vi "DAQ_Readings_from_DVS_plotting_and_saving.vi"() -> ()   [LabVIEW 2013]
uses:
  <vilib>/DAQmx/read.llb/DAQmx Read (Analog DBL 1Chan 1Samp).vi
  <vilib>/Utility/file.llb/Write To Spreadsheet File (string).vi
  <vilib>/DAQmx/miscellaneous.llb/DAQmx Fill In Error Info.vi
panel:
  out "Waveform Chart":cluster{dbl, dbl, dbl, dbl, dbl}(graph)
  in  "stop":bool
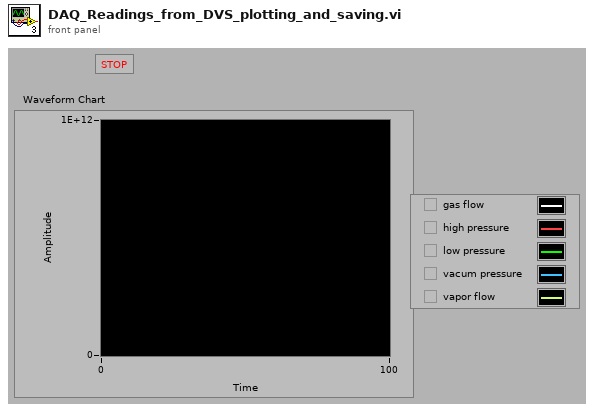
[diagram p1: front panel]
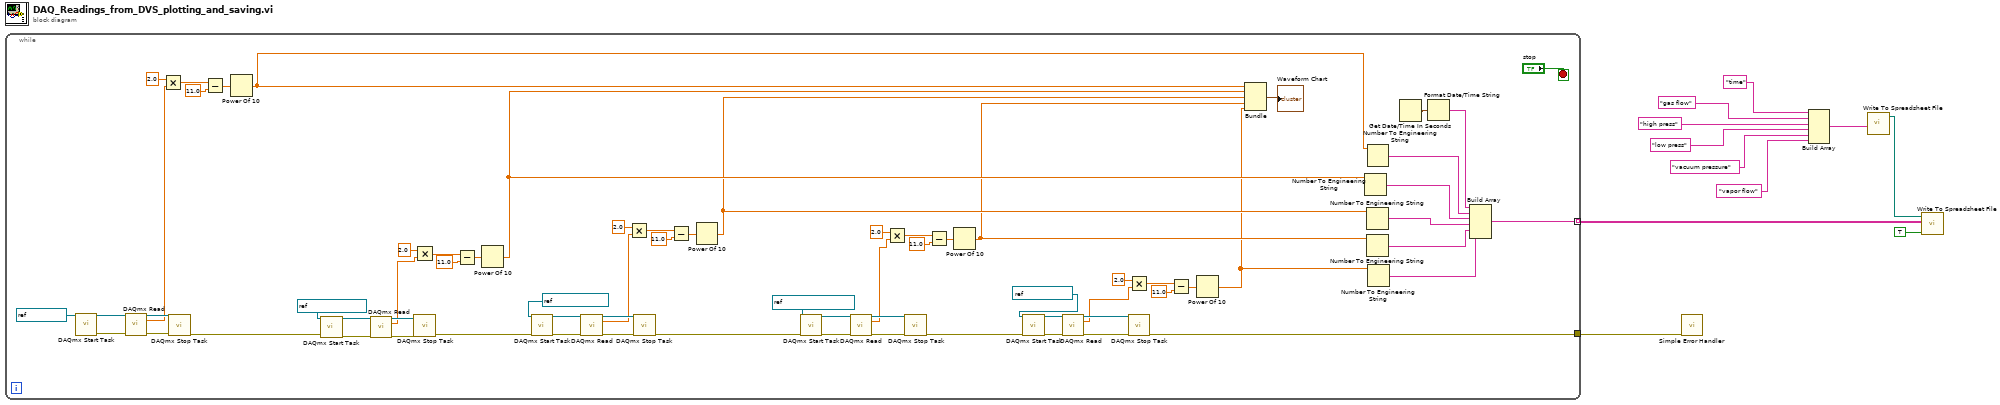
[diagram p0: block diagram]
diagram:
  n1 = while {
    tunnel: [w49] -> w1
    tunnel: [w24] -> w2 mode=indexing
    stop <- "stop" stop-if-true
    n2 = call <vilib>:"DAQmx Start Task.vi"("task/channels in"=refnum<k21> "GasFlow") -> ("task out"=w76:refnum<k21>, "error out"=w73:errorcluster)  [unwired: 13 in]
    n3 = call-poly <vilib>:"DAQmx Read.vi"("task/channels in"=w76, "error in"=w73) -> ("task out"=w75:refnum<k21>, "data"=w42:dbl, "error out"=w74:errorcluster)  [unwired: 11 in]
    n4 = Multiply(x=2.0, y=w42) -> (x*y=w44:dbl)
    n5 = call <vilib>:"DAQmx Stop Task.vi"("task/channels in"=w75, "error in"=w74) -> ("error out"=w52:errorcluster)  [unwired: 12 in, 1 out]
    n6 = Subtract(x=w44, y=11.0) -> (x-y=w46:dbl)
    n7 = Power Of 10(x=w46) -> (10^x=w22:dbl)
    n8 = call <vilib>:"DAQmx Start Task.vi"("task/channels in"=refnum<k21> "HighPressure", "error in"=w52) -> ("task out"=w72:refnum<k21>, "error out"=w69:errorcluster)  [unwired: 12 in]
    n9 = call-poly <vilib>:"DAQmx Read.vi"("task/channels in"=w72, "error in"=w69) -> ("task out"=w71:refnum<k21>, "data"=w37:dbl, "error out"=w70:errorcluster)  [unwired: 11 in]
    n10 = Multiply(x=2.0, y=w37) -> (x*y=w39:dbl)
    n11 = call <vilib>:"DAQmx Stop Task.vi"("task/channels in"=w71, "error in"=w70) -> ("error out"=w25:errorcluster)  [unwired: 12 in, 1 out]
    n12 = Subtract(x=w39, y=11.0) -> (x-y=w41:dbl)
    n13 = Power Of 10(x=w41) -> (10^x=w21:dbl)
    n14 = call <vilib>:"DAQmx Start Task.vi"("task/channels in"=refnum<k21> "LowPressure", "error in"=w25) -> ("task out"=w66:refnum<k21>, "error out"=w63:errorcluster)  [unwired: 12 in]
    n15 = call-poly <vilib>:"DAQmx Read.vi"("task/channels in"=w66, "error in"=w63) -> ("task out"=w65:refnum<k21>, "data"=w32:dbl, "error out"=w64:errorcluster)  [unwired: 11 in]
    n16 = Multiply(x=2.0, y=w32) -> (x*y=w34:dbl)
    n17 = call <vilib>:"DAQmx Stop Task.vi"("task/channels in"=w65, "error in"=w64) -> ("error out"=w51:errorcluster)  [unwired: 12 in, 1 out]
    n18 = Subtract(x=w34, y=11.0) -> (x-y=w36:dbl)
    n19 = Power Of 10(x=w36) -> (10^x=w20:dbl)
    n20 = call <vilib>:"DAQmx Start Task.vi"("task/channels in"=refnum<k21> "VacuumPressure", "error in"=w51) -> ("task out"=w62:refnum<k21>, "error out"=w59:errorcluster)  [unwired: 12 in]
    n21 = call-poly <vilib>:"DAQmx Read.vi"("task/channels in"=w62, "error in"=w59) -> ("task out"=w61:refnum<k21>, "data"=w27:dbl, "error out"=w60:errorcluster)  [unwired: 11 in]
    n22 = Multiply(x=2.0, y=w27) -> (x*y=w29:dbl)
    n23 = call <vilib>:"DAQmx Stop Task.vi"("task/channels in"=w61, "error in"=w60) -> ("error out"=w50:errorcluster)  [unwired: 12 in, 1 out]
    n24 = Subtract(x=w29, y=11.0) -> (x-y=w31:dbl)
    n25 = Power Of 10(x=w31) -> (10^x=w19:dbl)
    n26 = call <vilib>:"DAQmx Start Task.vi"("task/channels in"=refnum<k21> "VaporFlow", "error in"=w50) -> ("task out"=w53:refnum<k21>, "error out"=w56:errorcluster)  [unwired: 12 in]
    n27 = call-poly <vilib>:"DAQmx Read.vi"("task/channels in"=w53, "error in"=w56) -> ("task out"=w54:refnum<k21>, "data"=w26:dbl, "error out"=w55:errorcluster)  [unwired: 11 in]
    n28 = Multiply(x=2.0, y=w26) -> (x*y=w78:dbl)
    n29 = call <vilib>:"DAQmx Stop Task.vi"("task/channels in"=w54, "error in"=w55) -> ("error out"=w49:errorcluster)  [unwired: 12 in, 1 out]
    n30 = Subtract(x=w78, y=11.0) -> (x-y=w80:dbl)
    n31 = Power Of 10(x=w80) -> (10^x=w18:dbl)
    n32 = Bundle(w22, w21, w20, w19, w18) -> (→"Waveform Chart":cluster{dbl, dbl, dbl, dbl, dbl})  [unwired: 1 in]
    n33 = Number To Engineering String(4:w21) -> (0:w16:string)  [unwired: 3 in]
    n34 = Number To Engineering String(4:w20) -> (0:w15:string)  [unwired: 3 in]
    n35 = Number To Engineering String(4:w19) -> (0:w14:string)  [unwired: 3 in]
    n36 = Number To Engineering String(4:w22) -> (0:w17:string)  [unwired: 3 in]
    n37 = Number To Engineering String(4:w18) -> (0:w13:string)  [unwired: 3 in]
    n38 = Get Date/Time In Seconds() -> (seconds since 1Jan1904=w81:timestamp)
    n39 = Format Date/Time String(seconds (now)=w81) -> (date/time string=w23:string)  [unwired: 2 in]
    n40 = Build Array(w23, w17, w16, w15, w14, w13) -> (w24:string[])
  }
  n41 = call <vilib>:"Simple Error Handler.vi"("error in (no error)"=w1) -> ()  [unwired: 4 in, 5 out]
  n42 = Build Array("time", "gas flow", "high press", "low press" ("element"), "vacuum pressure" ("element"), "vapor flow" ("element")) -> (w8:string[])
  n43 = call-poly <vilib>:"Write To Spreadsheet File.vi"("1D data"=w8) -> ("new file path (Not A Path if cancelled)"=w7:path)  [unwired: 7 in]
  n44 = call-poly <vilib>:"Write To Spreadsheet File.vi"("append to file? (new file:F)"=TRUE, "2D data"=w2, "file path (dialog if empty)"=w7) -> ()  [unwired: 5 in, 1 out]
